vi "Actor Core.vi"(8 "error in":errorcluster, 11 "Cursor Digitizer in":refnum<class "Cursor Digitizer.lvclass">) -> (0 "error out":errorcluster, 3 "Actor out":refnum<class "Actor.lvclass">)   [LabVIEW 2016, in "Cursor Digitizer.lvclass"]
doc: "(<B>Filename</B>: Actor Framework.lvlib:Actor.lvclass:Actor Core.vi)\n\nReceives messages to the actor, reacts to them, and initiates any error handling that may shut the actor down.\n\nDescendant classes may override this VI to append parallel tasks for the actor to complete while it handles messages. Overrides use the Call Parent Method node."
uses:
  Cursor Digitizer.lvclass
  Cursor Digitizer Messages/Update Cursor State Msg/Update Cursor State Msg.lvclass
  <vilib>/ActorFramework/Actor/Actor.lvclass
  <vilib>/event_ctls.llb/eventvkey.ctl
  Cursor Digitizer Messages/Store XY Msg/Store XY Msg.lvclass
  <vilib>/Utility/file.llb/Write Delimited Spreadsheet (DBL).vi
  Template Module/Template Module.lvclass
  C:/Program Files (x86)/National Instruments/LabVIEW 2016/vi.lib/ActorFramework/Actor/Actor.lvclass
panel:
  in  "Clear Button":bool
  in  "Save Button":bool
  in  "X-Y values":dbl[][](array[numeric]) format="%#_6p"
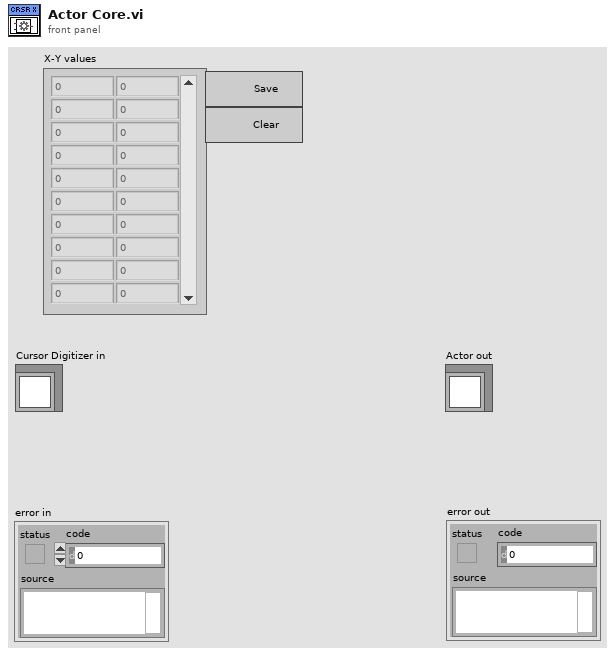
[diagram p1: front panel]
types:
  T1 = typedef "eventvkey.ctl" = enum16{"ASCII", "Enter", "Return", "Shift", "Ctrl", "Alt", "Cmd", "Opt", "Caps", "NumLock", "Clear", "Break", "Up", "Down", "Left", "Right", "Insert", "Delete", "Home", "End", "PageUp", "PageDown", "Escape", "Help", "Pause", "ScrollLock", "F1", "F2", "F3", "F4", "F5", "F6", "F7", "F8", "F9", "F10", "F11", "F12", "F13", "F14", "F15", "F16", "F17", "F18", "F19", "F20", "F21", "F22", "F23", "F24", "Play", "VolumeUp", "VolumeDown", "Mute", "Two Byte Char"}
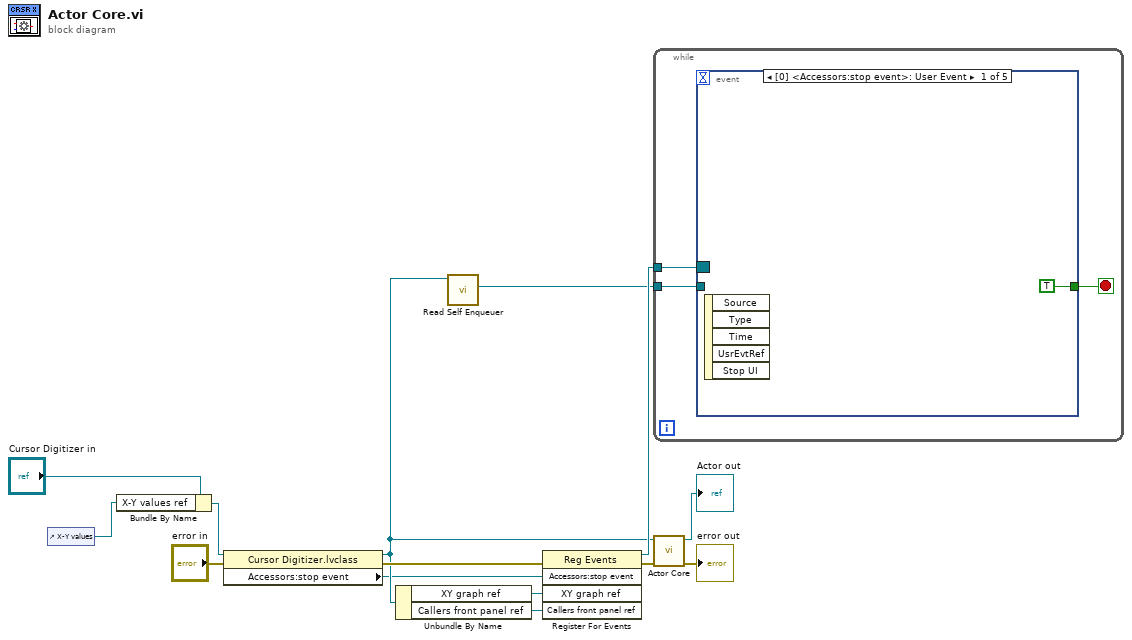
[diagram p0: block diagram]
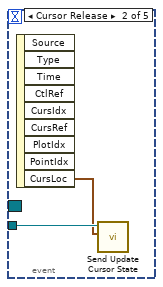
[diagram p2: hidden frame]
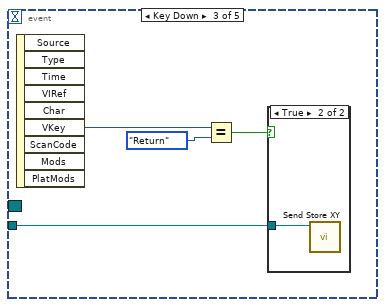
[diagram p3: hidden frame]
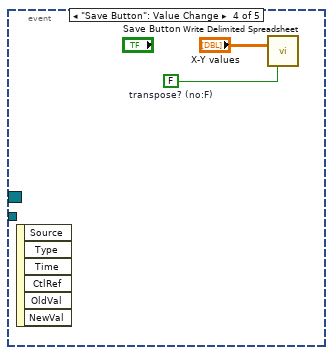
[diagram p5: hidden frame]
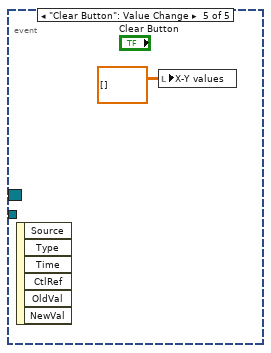
[diagram p6: hidden frame]
diagram:
  n1 = control-ref of="X-Y values"() -> (w5:refnum<vi>)
  n2 = Bundle By Name(cluster="Cursor Digitizer in", "X-Y values ref"=w5) -> (w3:refnum<class "Cursor Digitizer.lvclass">)
  n3 = property class="Cursor Digitizer.lvclass"(reference=w3, error in="error in") -> (reference out=w2:refnum<class "Cursor Digitizer.lvclass">, error out=w4:errorcluster, "Accessors:stop event"=w1:refnum<user-event>)
  n4 = Unbundle By Name(w2) -> ("XY graph ref"=w7:refnum<vi>, "Callers front panel ref"=w6:refnum<vi>)
  n5 = call <vilib>:"Read Self Enqueuer.vi"("Actor"=w2) -> ("Self Enqueuer"=w8:refnum<class "Message Enqueuer.lvclass">)  [unwired: 10 in]
  n6 = register-events(error in=w4, w1, w7, w6) -> (reference out=w10:refnum<event-registration>, error out=w11:errorcluster)  [unwired: 1 in]
  n7 = while {
    tunnel: w10 -> [w17]
    tunnel: w8 -> [w15]
    stop <- w16 stop-if-true
    n8 = event shown="[0] <Accessors:stop event>: User Event" {
      selector: w17 -> [_ _ _ _ _]
      dyn-events: _ -> [_ _ _ _ _]
      timeout: _ -> [_ _ _ _ _]
      tunnel: [TRUE _ _ _ _] -> w16
      tunnel: w15 -> [_ w20 w21 _ _]
      event User Event {
        n9 = event-data() -> ()  [unwired: 1 in, 5 out]
      }
      event Cursor Release {
        n10 = event-data() -> ("CursLoc"=w19:cluster{"X":dbl, "Y":dbl})  [unwired: 1 in, 8 out]
        n11 = call "Send Update Cursor State.vi"("Cursor State"=w19, "Message Enqueuer"=w20) -> ()  [unwired: 8 in, 2 out]
      }
      event Key Down {
        n12 = event-data() -> ("VKey"=w24:T1)  [unwired: 1 in, 8 out]
        n13 = Equal?(x=w24, y=eventvkey."Return" ("VKey")) -> (x = y?=w22:bool)
        n14 = case shown="True" w22 {
          tunnel: w21 -> [_ w25]
          frame False {
          }
          frame True {
            n15 = call "Send Store XY.vi"("Message Enqueuer"=w25) -> ()  [unwired: 9 in, 2 out]
          }
        }
      }
      event "Save Button": Value Change {
        w26 = FALSE  # transpose? (no:F)
        n16 = event-data() -> ()  [unwired: 1 in, 6 out]
        n17 = call-poly <vilib>:"Write Delimited Spreadsheet.vi"("2D data"="X-Y values", "transpose? (no:F)"=w26) -> ()  [unwired: 12 in, 2 out]
      }
      event "Clear Button": Value Change {
        n18 = event-data() -> ()  [unwired: 1 in, 6 out]
        n19 = local write "X-Y values"(dbl[][] [] ("X-Y values")) -> ()
      }
    }
  }
  n20 = call-parent "Actor Core.vi"("error in"=w11, "Measure Object in"=w2) -> ("error out"=→"error out":errorcluster, "Actor out"=→"Actor out":refnum<class "Actor.lvclass">)  [unwired: 8 in]
